vi "continue.vi"(8 "error in":errorcluster) -> (3 "continue?":bool)   [LabVIEW 2012]
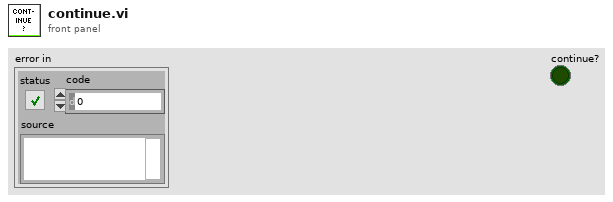
[diagram p1: front panel]
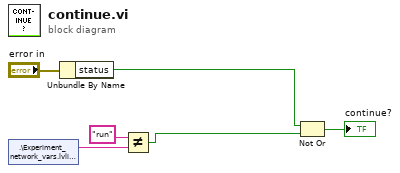
[diagram p0: block diagram]
diagram:
  n1 = shared-variable ".\\Experiment_network_vars.lvlib\\state"() -> (w6:string)  [unwired: 1 in, 1 out]
  n2 = Unbundle By Name("error in") -> ("status"=w3:bool)
  n3 = Not Equal?(x="run", y=w6) -> (x != y?=w2:bool)
  n4 = Not Or(1:w2, 2:w3) -> (0:→"continue?":bool)
